vi "Configure Acquisition.vi"(8 "error in (no error)":errorcluster, 11 "object in":refnum<class "Fetch Waveforms CFG.lvclass">) -> (0 "error out":errorcluster, 3 "object out":refnum<class "Fetch Waveforms CFG.lvclass">)   [LabVIEW 2023, in "Scope Simulated CFGs.lvlib" / "Fetch Waveforms CFG.lvclass"]
uses:
  Fetch Waveforms CFG.lvclass
  D:/git/HAL/HAL GOOP4/Configuration/Configuration JSON/Configuration JSON Base/CFG JSON.lvclass
  Configuration/Configuration JSON/Configuration JSON Base/CFG JSON.lvclass/CFG JSON.ctl
  51f59c3a-b204-4edc-9e9c-c04e48498727.vi
  <vilib>/JDP Science/JSONtext/Find Item.vi
  <vilib>/JDP Science/JSONtext/Next JSON Value.vi
  <vilib>/JDP Science/JSONtext/String Subset.vi
  <vilib>/JDP Science/JSONtext/Parsing/Advance past next JSON Value (inlined COPY).vi
  <vilib>/JDP Science/JSONtext/Parsing/Advance past whitespace.vi
  <vilib>/JDP Science/JSONtext/Parsing/Advance past String.vi
  <vilib>/JDP Science/JSONtext/Parsing/Advance past Number.vi
  <vilib>/JDP Science/JSONtext/Parsing/Advance past Line Ending.vi
  <vilib>/JDP Science/JSONtext/Parsing/Parse Full Path or Item Name.vi
  <vilib>/JDP Science/JSONtext/Parsing/Advance past Array.vi
  <vilib>/JDP Science/JSONtext/Parsing/Advance past Object.vi
  <vilib>/JDP Science/JSONtext/support/Error Cluster From Code.vi
  <vilib>/JDP Science/JSONtext/Offset/Find Item Locations by Path.vi
  <vilib>/JDP Science/JSONtext/JSON text to Variant.vi
  <vilib>/Utility/error.llb/Error Cluster From Error Code.vi
  <vilib>/JDP Science/JSONtext/LVClass Serializer/JSONtext LVClass Serializer.lvclass
  <vilib>/ErrorRing/Error Ring.xnode
  Configuration/Configuration JSON/Configuration JSON Base/CFG JSON.lvclass
panel:
  out "Data":T1
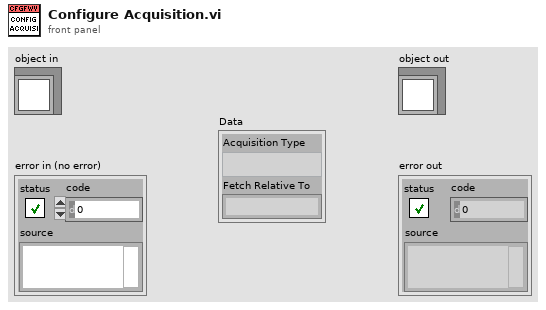
[diagram p1: front panel]
types:
  T1 = cluster{"Type":string, "Fetch Relative To":string}
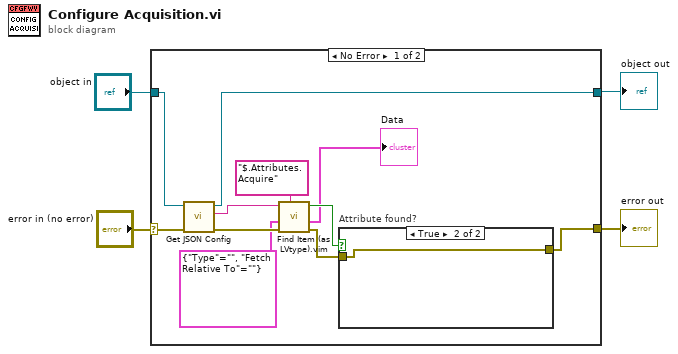
[diagram p0: block diagram]
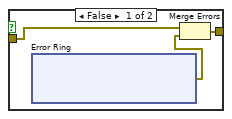
[diagram p2: hidden frame]
diagram:
  n1 = case shown="No Error" "error in (no error)" {
    selector: "error in (no error)" -> [w14 w26]
    tunnel: [w6 w26] -> w3
    tunnel: [w11 w25] -> w1
    tunnel: "object in" -> [w12 w25]
    frame No Error {
      n2 = call "Get JSON Config.vi"("error in (no error)"=w14, "CFG Base in"=w12) -> ("error out"=w13:errorcluster, "<JSON>Config>"=w10:string, "CFG Base out"=w11:refnum<class "Fetch Waveforms CFG.lvclass">)  [unwired: 7 in]
      n3 = call "Find Item (as LVtype).vim"("$Path or Item Name"="$.Attributes.Acquire", "error in (no error)"=w13, "Data Type and Default Value"=T1 {"Type"="", "Fetch Relative To"=""}, "JSON"=w10) -> ("error out"=w7:errorcluster, "Data"=→"Data":T1, "Found"=w8:bool)  [unwired: 4 in, 1 out]
      n4 = case "Attribute found?" shown="True" w8 {
        tunnel: w7 -> [w18 w24]
        tunnel: [w16 w24] -> w6
        frame False {
          n5 = xnode "Error Ring"() -> ("error out"=w17:errorcluster)
          n6 = Merge Errors(w18, w17) -> (w16:errorcluster)
        }
        frame True {
        }
      }
    }
    frame Error {
    }
  }
  "error out" <- w3
  "object out" <- w1
